vi "Compute Distance.vi"(9 "X Image Resolution":i32, 10 "Bounding Box":T1, 11 "Camera Type":enum16{"206", "1011"}(ring)) -> (2 "Target Center":cluster{"X":dbl, "Y":dbl}, 3 "Distance (ft)":dbl)   [LabVIEW 2011]
doc: "Using the camera lens information and the real world width of the target, determine the distance to the target."
panel:
  in  "Camera view angle":dbl[](array[numeric])=[48.0, 43.5]
  # "Axis 206\nAxis M1011"
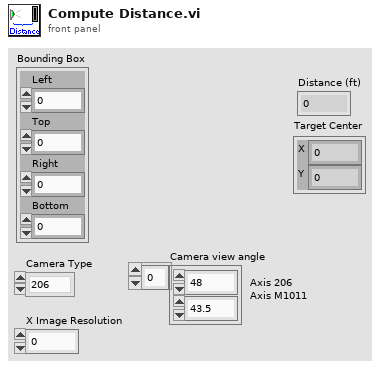
[diagram p1: front panel]
types:
  T1 = cluster{"Left":dbl, "Top":dbl, "Right":dbl, "Bottom":dbl}
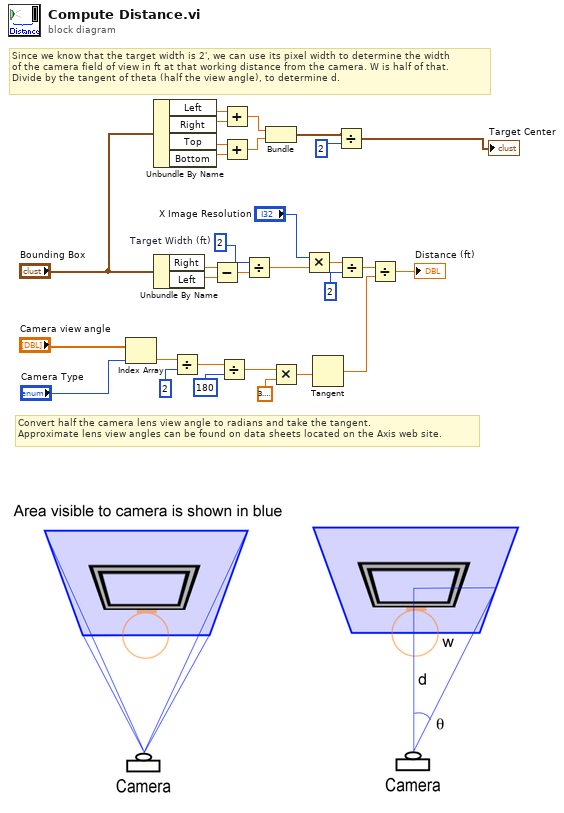
[diagram p0: block diagram]
diagram:
  w12 = 2  # Target Width (ft)
  # "Convert half the camera lens view angle to radians and take the tangent.\nApproximate lens view angles can be found on data sheets located on the Axis web site."
  # "Since we know that the target width is 2', we can use its pixel width to determine the width\nof the camera field of view in ft at that working distance from the camera. W is half of that.\nDivide by the tangent of theta (half the view angle), to determine d."
  n1 = Index Array(array="Camera view angle", index="Camera Type") -> (element=w26:dbl)
  n2 = Unbundle By Name("Bounding Box") -> ("Left"=w7:dbl, "Right"=w8:dbl, "Top"=w10:dbl, "Bottom"=w9:dbl)
  n3 = Unbundle By Name("Bounding Box") -> ("Right"=w16:dbl, "Left"=w15:dbl)
  n4 = Divide(x=w26, y=2) -> (x/y=w23:dbl)
  n5 = Subtract(x=w16, y=w15) -> (x-y=w14:dbl)
  n6 = Divide(x=w23, y=180) -> (x/y=w22:dbl)
  n7 = Add(x=w7, y=w8) -> (x+y=w6:dbl)
  n8 = Add(x=w10, y=w9) -> (x+y=w5:dbl)
  n9 = Divide(x=w12, y=w14) -> (x/y=w13:dbl)
  n10 = Bundle(w6, w5) -> (w2:cluster{dbl, dbl})  [unwired: 1 in]
  n11 = Multiply(x=w22, y=3.141592653589793) -> (x*y=w24:dbl)
  n12 = Multiply(x="X Image Resolution", y=w13) -> (x*y=w17:dbl)
  n13 = Tangent(1:w24) -> (0:w30:dbl)
  n14 = Divide(x=w2, y=2) -> (x/y=→"Target Center":cluster{dbl, dbl})
  n15 = Divide(x=w17, y=2) -> (x/y=w19:dbl)
  n16 = Divide(x=w19, y=w30) -> (x/y=→"Distance (ft)":dbl)
